vi "new_neuron.vi"(8 "Offset":fxp<+/-,64,32>, 10 "Weights":fxp<+/-,64,32>[](array[numeric]), 11 "Inputs":fxp<+/-,64,32>[](array[numeric])) -> (3 "Output":fxp<+/-,64,32>)   [LabVIEW 2014]
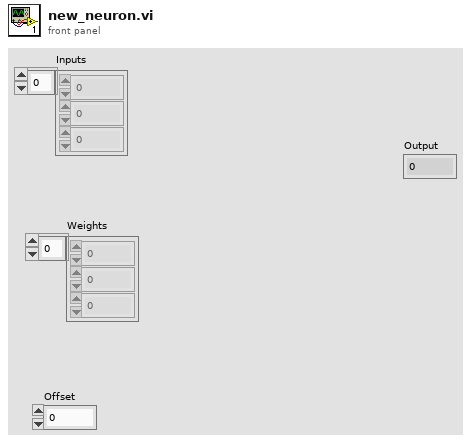
[diagram p1: front panel]
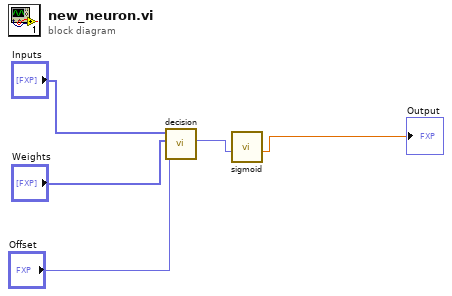
[diagram p0: block diagram]
diagram:
  n1 = call "decision.vi"("offset"="Offset", "weights"="Weights", "inputs"="Inputs") -> ("decision"=w5:fxp<+/-,64,32>)  [unwired: 8 in]
  n2 = call "sigmoid.vi"("t"=w5) -> ("S(t)"=→"Output":dbl)  [unwired: 10 in]
